vi "OCUMain.vi"() -> ()   [LabVIEW 2014]
uses:
  Command.ctl
  DataHighway.ctl
  P:/+Courses/ENGR_3390_Robotics_I/ENGR3390_Fall_2015/For Justin/Project 5 Act Lab Code 2015/Command.ctl
  P:/+Courses/ENGR_3390_Robotics_I/ENGR3390_Fall_2015/For Justin/Project 5 Act Lab Code 2015/DataHighway.ctl
  <vilib>/ErrorRing/Error Ring.xnode
panel:
  out "DataHWay":T1
  out "ComHWay":T2 {"Speed" scale=-2.0..10.0; "Rudder" scale=-10.0..10.0}
  out "OCU Running":bool
  out "Tab Control":T3(tab)
  out "Starboard":dbl(slide) scale=0.0..80.0
  out "Front":dbl(slide) scale=0.0..80.0
  out "Boolean 5":bool
  out "Boolean 4":bool
  out "Boolean 3":bool
  out "Boolean 2":bool
  out "Boolean":bool
  in  "Beh Lights ok?":bool
  in  "myRIO ok?":bool
  in  "Prop ok?":bool
  in  "Rudder ok?":bool
  in  "Sharp IR-Lidar ok?":bool
  in  "Goto Debug?":bool
  out "MyRIO":bool
  out "Port":dbl(slide)
  in  "Re-Initialize":bool
  in  "Debug Robot":bool
  in  "Run Robot":bool
  in  "Stop OCU":bool
  out "Sharp IR Lidar":T4(graph)
  in  "Debug Complete?":bool
  out "RobotRunning":bool
  out "HW-Stop":bool
  in  "E-Stop Motors":bool
  in  "Exit Run":bool
  # "Press Arrow\nabove to start\nOCU running"
  # "Run auto Initialize sequence.\nIndicate which functionality is ok.\nAll functions must work or choose go to debug state."
  # "Look at boat?"
  # "Look at boat?"
  # "Look at boat?"
  # "Unit Test"
  # "Function"
  # "Press button to\nselect robot state"
  # "Robot Initialized and \nwaiting for user input"
  # "OCU and Robot safely shut down"
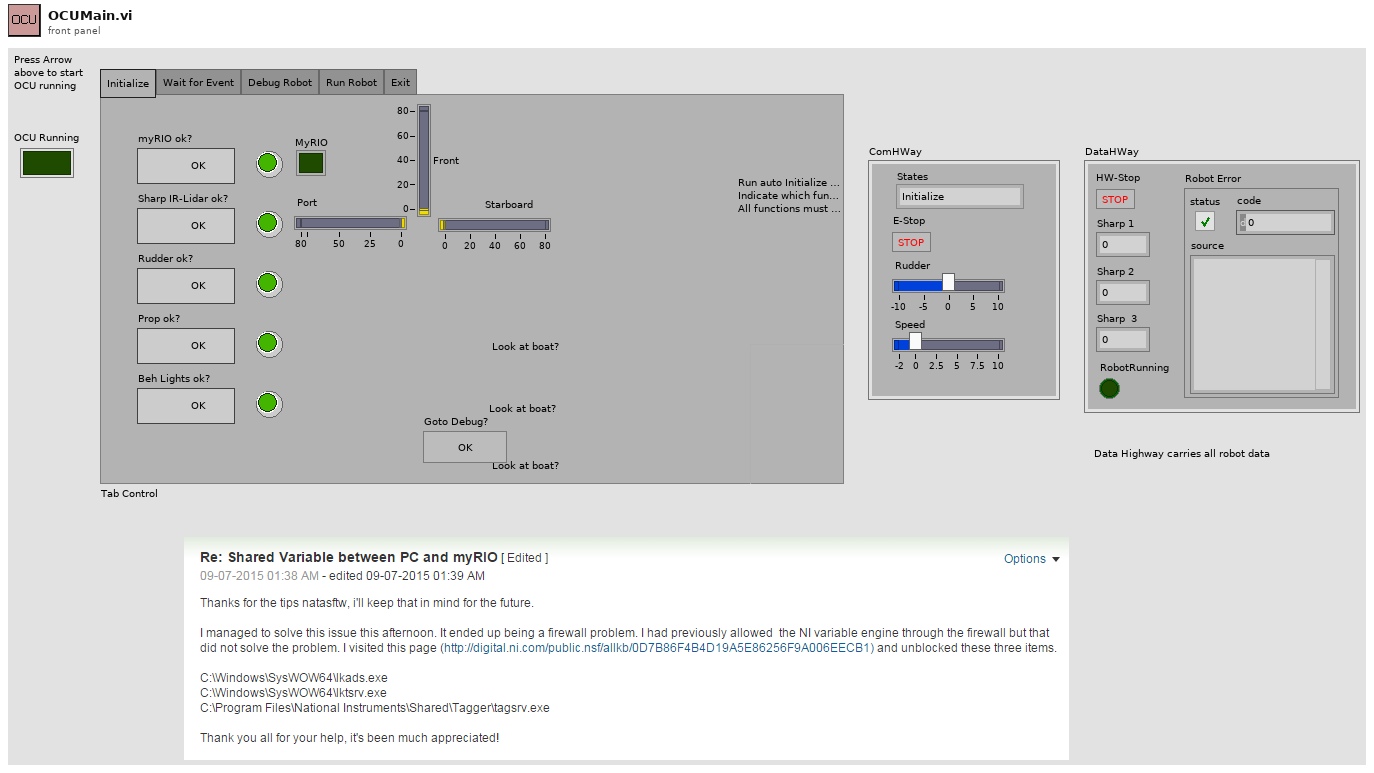
[diagram p1: front panel]
types:
  T1 = typedef "DataHighway.ctl" = cluster{"HW-Stop":bool, "Sharp 1":dbl, "Sharp 2":dbl, "Sharp  3":dbl, "RobotRunning":bool, "Robot Error":errorcluster}
  T2 = typedef "Command.ctl" = cluster{"States":enum16{"Initialize", "Wait for Event", "Debug Robot", "Run Robot", "Exit"}, "E-Stop":bool, "Rudder":dbl, "Speed":dbl}
  T3 = enum32{"Initialize", "Wait for Event", "Debug Robot", "Run Robot", "Exit"}
  T4 = cluster{"Sharp 1":dbl, "Sharp 2":dbl, "Sharp  3":dbl}
  T5 = enum16{"Initialize", "Wait for Event", "Debug Robot", "Run Robot", "Exit"}
  T6 = cluster{"Port":dbl, "Center":dbl, "Starboard":dbl}
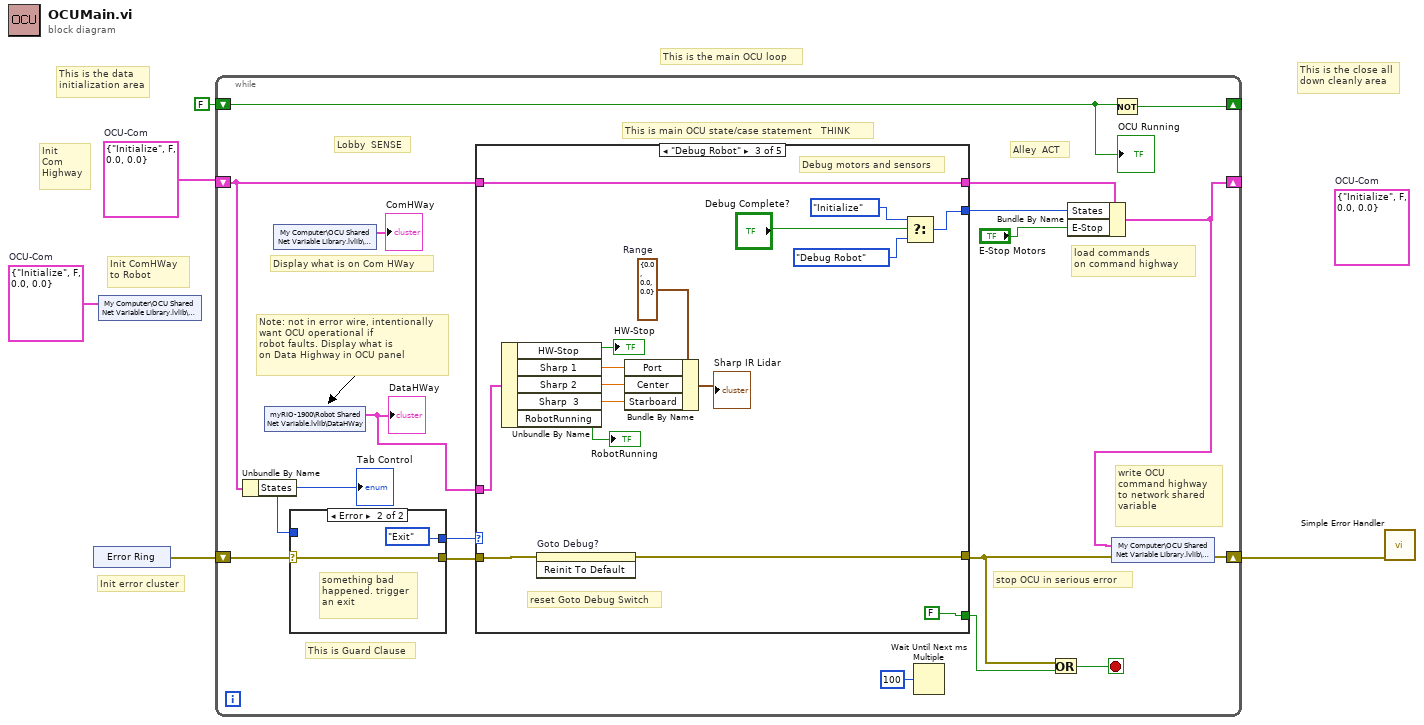
[diagram p0: block diagram]
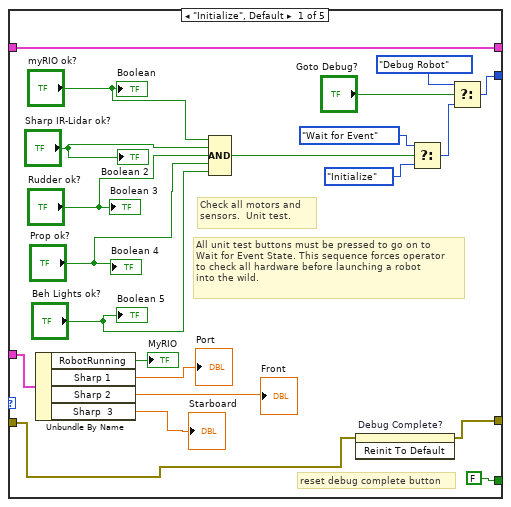
[diagram p3: hidden frame]
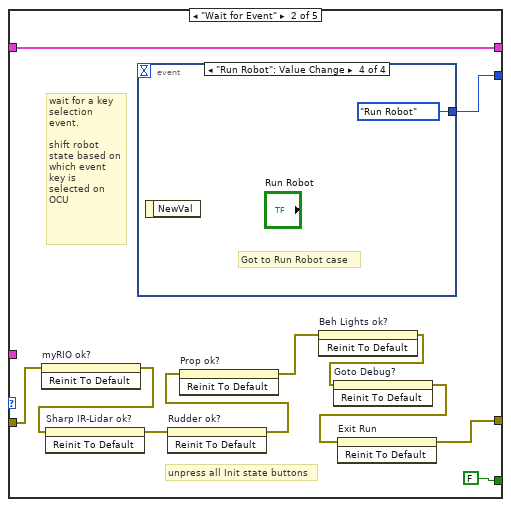
[diagram p4: hidden frame]
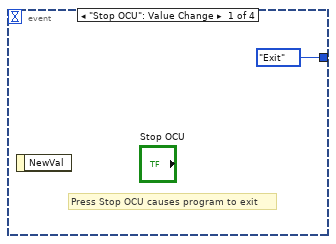
[diagram p5: hidden frame]
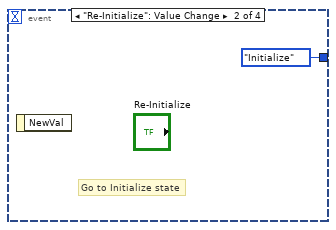
[diagram p6: hidden frame]
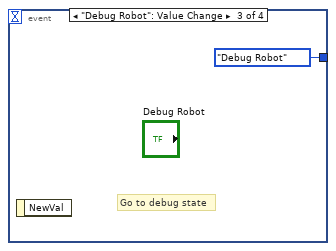
[diagram p7: hidden frame]
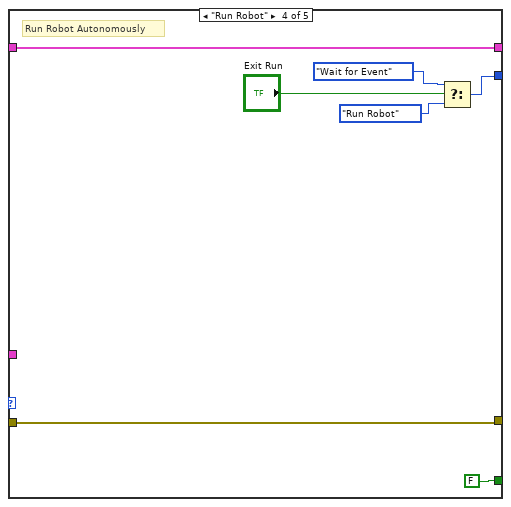
[diagram p8: hidden frame]
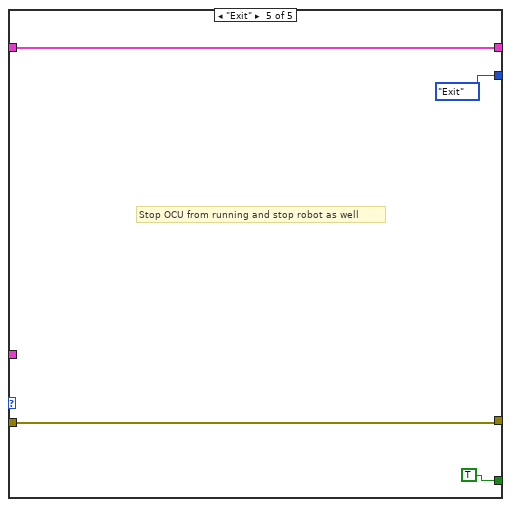
[diagram p9: hidden frame]
diagram:
  (unwired) T2 {"States"=enum."Initialize", "E-Stop"=FALSE, "Rudder"=0.0, "Speed"=0.0}  # OCU-Com
  w1 = T2 {"States"=enum."Initialize", "E-Stop"=FALSE, "Rudder"=0.0, "Speed"=0.0}  # OCU-Com
  w2 = T2 {"States"=enum."Initialize", "E-Stop"=FALSE, "Rudder"=0.0, "Speed"=0.0}  # OCU-Com
  # "Init ComHWay\nto Robot"
  # "Init error cluster"
  # "Init\nCom\nHighway"
  # "This is the close all\ndown cleanly area"
  # "This is the data\ninitialization area"
  # "This is the main OCU loop"
  n1 = xnode "Error Ring"() -> ("error out"=w4:errorcluster)
  n2 = shared-variable "My Computer\\OCU Shared Net Variable Library.lvlib\\ComHWay"(w1) -> ()  [unwired: 1 in, 1 out]
  n3 = while {
    shift-right: [w22] -> _
    shift-left: FALSE -> [w21]
    shift-right: [w11] -> w3
    shift-left: w4 -> [w20]
    shift-right: [w7] -> _
    shift-left: w2 -> [w15]
    stop <- w17 stop-if-true
    # "Note: not in error wire, intentionally\nwant OCU operational if\nrobot faults. Display what is \non Data Highway in OCU panel"
    # "load commands\non command highway"
    # "Display what is on Com HWay"
    # "write OCU  \ncommand highway\nto network shared\nvariable"
    # "stop OCU in serious error"
    # "This is Guard Clause"
    # "This is main OCU state/case statement   THINK"
    # "Alley  ACT"
    # "Lobby  SENSE"
    n4 = Unbundle By Name "Unbundle By Name"(w15) -> ("States"=w14:T5)
    "Tab Control" <- w14
    n5 = shared-variable "myRIO-1900\\Robot Shared Net Variable.lvlib\\DataHWay"() -> (w6:T1)  [unwired: 1 in, 1 out]
    "DataHWay" <- w6
    n6 = shared-variable "My Computer\\OCU Shared Net Variable Library.lvlib\\ComHWay"() -> (→"ComHWay":T2)  [unwired: 1 in, 1 out]
    n7 = case shown="Error" w20 {
      selector: w20 -> [w25 w27]
      tunnel: [w25 w27] -> w19
      tunnel: w14 -> [w24 _]
      tunnel: [w24 T5."Exit" ("States")] -> w16
      frame No Error {
      }
      frame Error {
        # "something bad\nhappened. trigger\nan exit"
      }
    }
    n8 = case shown="\"Debug Robot\"" w16 {
      tunnel: [w47 w58 w77 w84 T5."Exit" ("States")] -> w13
      tunnel: [FALSE FALSE FALSE FALSE TRUE] -> w18
      tunnel: w19 -> [w32 w57 w74 w82 w88]
      tunnel: [w35 w49 w73 w82 w88] -> w12
      tunnel: w15 -> [w34 w51 w72 w80 w87]
      tunnel: [w34 w51 w72 w80 w87] -> w10
      tunnel: w6 -> [w33 _ w71 _ _]
      frame "Initialize", Default {
        # "reset debug complete button"
        # "All unit test buttons must be pressed to go on to \nWait for Event State. This sequence forces operator\nto check all hardware before launching a robot\ninto the wild."
        # "Check all motors and \nsensors.  Unit test."
        n9 = Unbundle By Name(w33) -> ("RobotRunning"=→"MyRIO":bool, "Sharp 1"=→"Port":dbl, "Sharp 2"=→"Front":dbl, "Sharp  3"=→"Starboard":dbl)
        n10 = Compound Arithmetic op=AND("myRIO ok?", "Sharp IR-Lidar ok?", "Rudder ok?", "Prop ok?", "Beh Lights ok?") -> (w36:bool)
        n11 = invoke on="Debug Complete?" class="Bool (strict)" method="Reinit To Default"(error in=w32) -> (error out=w35:errorcluster)  [unwired: 2 in, 2 out]
        n12 = Select ("Select next state")(t=T5."Wait for Event" ("States"), s=w36, f=T5."Initialize") -> (s? t:f=w44:T5)
        n13 = Select ("Select next state")(t=T5."Debug Robot" ("f"), s="Goto Debug?", f=w44) -> (s? t:f=w47:T5)
        "Boolean" <- "myRIO ok?"
        "Boolean 2" <- "Sharp IR-Lidar ok?"
        "Boolean 3" <- "Rudder ok?"
        "Boolean 4" <- "Prop ok?"
        "Boolean 5" <- "Beh Lights ok?"
      }
      frame "Wait for Event" {
        # "unpress all Init state buttons"
        # "wait for a key \nselection\nevent.\n\nshift robot\nstate based on\nwhich event\nkey is\nselected on \nOCU"
        n14 = invoke on="myRIO ok?" class="Bool (strict)" method="Reinit To Default"(error in=w57) -> (error out=w56:errorcluster)  [unwired: 2 in, 2 out]
        n15 = invoke on="Sharp IR-Lidar ok?" class="Bool (strict)" method="Reinit To Default"(error in=w56) -> (error out=w55:errorcluster)  [unwired: 2 in, 2 out]
        n16 = event shown="[3] \"Run Robot\": Value Change" {
          selector: _ -> [_ _ _ _]
          dyn-events: _ -> [_ _ _ _]
          timeout: _ -> [_ _ _ _]
          tunnel: [T5."Exit" ("States") T5."Initialize" ("States") T5."Debug Robot" ("States") T5."Run Robot" ("States")] -> w58
          event "Stop OCU": Value Change {
            # "Press Stop OCU causes program to exit"
            n17 = event-data() -> ()  [unwired: 1 in, 1 out]
          }
          event "Re-Initialize": Value Change {
            # "Go to Initialize state"
            n18 = event-data() -> ()  [unwired: 1 in, 1 out]
          }
          event "Debug Robot": Value Change {
            # "Go to debug state"
            n19 = event-data() -> ()  [unwired: 1 in, 1 out]
          }
          event "Run Robot": Value Change {
            # "Got to Run Robot case"
            n20 = event-data() -> ()  [unwired: 1 in, 1 out]
          }
        }
        n21 = invoke on="Rudder ok?" class="Bool (strict)" method="Reinit To Default"(error in=w55) -> (error out=w54:errorcluster)  [unwired: 2 in, 2 out]
        n22 = invoke on="Prop ok?" class="Bool (strict)" method="Reinit To Default"(error in=w54) -> (error out=w53:errorcluster)  [unwired: 2 in, 2 out]
        n23 = invoke on="Beh Lights ok?" class="Bool (strict)" method="Reinit To Default"(error in=w53) -> (error out=w52:errorcluster)  [unwired: 2 in, 2 out]
        n24 = invoke on="Goto Debug?" class="Bool (strict)" method="Reinit To Default"(error in=w52) -> (error out=w50:errorcluster)  [unwired: 2 in, 2 out]
        n25 = invoke on="Exit Run" class="Bool (strict)" method="Reinit To Default"(error in=w50) -> (error out=w49:errorcluster)  [unwired: 2 in, 2 out]
      }
      frame "Debug Robot" {
        w65 = T6 {"Port"=0.0, "Center"=0.0, "Starboard"=0.0}  # Range
        # "reset Goto Debug Switch"
        # "Debug motors and sensors"
        n26 = Unbundle By Name "Unbundle By Name"(w71) -> ("HW-Stop"=→"HW-Stop":bool, "Sharp 1"=w68:dbl, "Sharp 2"=w67:dbl, "Sharp  3"=w66:dbl, "RobotRunning"=→"RobotRunning":bool)
        n27 = invoke on="Goto Debug?" class="Bool (strict)" method="Reinit To Default"(error in=w74) -> (error out=w73:errorcluster)  [unwired: 2 in, 2 out]
        n28 = Bundle By Name(cluster=w65, "Port"=w68, "Center"=w67, "Starboard"=w66) -> (→"Sharp IR Lidar":T6)
        n29 = Select(t=T5."Initialize" ("States"), s="Debug Complete?", f=T5."Debug Robot") -> (s? t:f=w77:T5)
      }
      frame "Run Robot" {
        # "Run Robot Autonomously"
        n30 = Select(t=T5."Wait for Event" ("States"), s="Exit Run", f=T5."Run Robot") -> (s? t:f=w84:T5)
      }
      frame "Exit" {
        # "Stop OCU from running and stop robot as well"
      }
    }
    n31 = Wait Until Next ms Multiple(millisecond multiple=u32 100) -> ()  [unwired: 1 out]
    n32 = Or(x=w12, y=w18) -> (x .or. y?=w17:bool)
    n33 = Bundle By Name(cluster=w10, "States"=w13, "E-Stop"="E-Stop Motors") -> (w7:T2)
    n34 = Not(x=w21) -> (.not. x?=w22:bool)
    n35 = shared-variable "My Computer\\OCU Shared Net Variable Library.lvlib\\ComHWay"(w7, error in=w12) -> (error out=w11:errorcluster)
    "OCU Running" <- w21
  }
  n36 = call <vilib>:"Simple Error Handler.vi"("error in (no error)"=w3) -> ()  [unwired: 4 in, 5 out]
